vi "Create_Trajectory_All_WP_Units_To_Meters.vi"(9 "Units Selector":T1, 11 "WayPoints":T2[](array[typedef]) {"WEIGHT" format="%13.3f"; "ANGLE" format="%13.3f"; "Y" format="%13.3f"; "X" format="%13.3f"}) -> (3 "Array":T2[](array[typedef]) {"WEIGHT" format="%13.3f"; "ANGLE" format="%13.3f"; "Y" format="%13.3f"; "X" format="%13.3f"})   [LabVIEW 2019]
uses:
  <vilib>/Rock Robotics/WPI/ThirdParty/JAS_Junk/TrajLib/TypeDef/DISPLAY_WEIGHTED_WAYPOINT.ctl
  CreateTrajectoryENUM/TrajCreateUnitsENUM.ctl
  <vilib>/Rock Robotics/WPI/ThirdParty/JAS_Junk/TrajLib/Conv_Inches_Meters.vi
  <vilib>/Rock Robotics/WPI/ThirdParty/JAS_Junk/TrajLib/Conv_Feet_Meters.vi
  <vilib>/Rock Robotics/WPI/ThirdParty/JAS_Junk/TrajLib/Trajectory_Library.lvlib
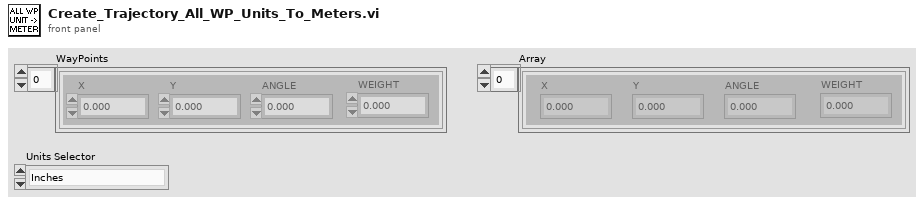
[diagram p1: front panel]
types:
  T1 = typedef "TrajCreateUnitsENUM.ctl" = enum16{"Inches", "Feet", "Centimeters", "Meters"}
  T2 = typedef "Trajectory_Library.lvlib/DISPLAY_WEIGHTED_WAYPOINT.ctl" = cluster{"X":dbl, "Y":dbl, "ANGLE":dbl, "WEIGHT":dbl}
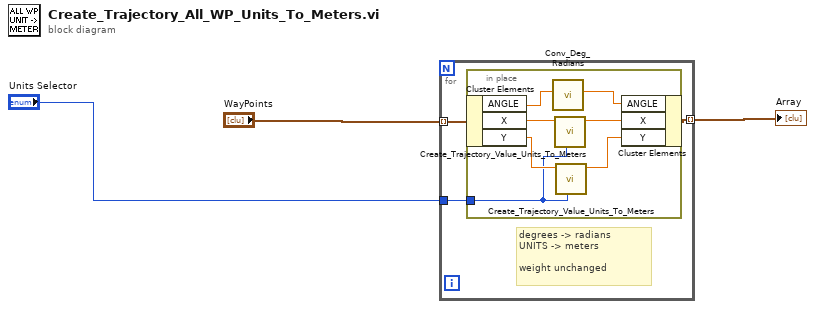
[diagram p0: block diagram]
diagram:
  n1 = for {
    tunnel: "WayPoints" -> [w6] mode=indexing
    tunnel: [w5] -> w2 mode=indexing
    tunnel: "Units Selector" -> [w4]
    # "degrees -> radians\nUNITS -> meters\n\nweight unchanged"
    n2 = in-place {
      in-place-border: w4 -> [w7]
      n3 = in-place-cluster #1(w6) -> ("ANGLE"=w8:dbl, "X"=w13:dbl, "Y"=w11:dbl)
      n4 = call <vilib>:"Conv_Deg_Radians.vi"("Degress"=w8) -> ("Radians"=w9:dbl)  [unwired: 10 in]
      n5 = call "Create_Trajectory_Value_Units_To_Meters.vi"("Units Selector"=w7, "Units"=w13) -> ("Meters"=w12:dbl)  [unwired: 9 in]
      n6 = call "Create_Trajectory_Value_Units_To_Meters.vi"("Units Selector"=w7, "Units"=w11) -> ("Meters"=w10:dbl)  [unwired: 9 in]
      n7 = in-place-cluster #1("ANGLE"=w9, "X"=w12, "Y"=w10) -> (w5:T2)
    }
  }
  "Array" <- w2
